vi "Set Timeout Trigger.vi"(8 "error in (no error)":errorcluster, 10 "Trigger Settings":T1, 11 "PXIe5105 in":refnum<class "PXIe5105.lvclass">) -> (0 "error out":errorcluster, 3 "PXIe5105 out":refnum<class "PXIe5105.lvclass">)   [LabVIEW 2018, in "PXIe5105.lvlib" / "PXIe5105.lvclass"]
doc: "This Override is used to configure a TimeOut Trigger."
uses:
  PXIe5105.lvclass
  PPLs/Oscilloscope/Parent/Oscilloscope.lvlibp/Custom Controls/Timeout Trigger Settings.ctl
  PPLs/Oscilloscope/Parent/Oscilloscope.lvlibp/Custom Controls/Analog Channels.ctl
  PPLs/Oscilloscope/Parent/Oscilloscope.lvlibp/Custom Controls/Trigger Mode.ctl
  PPLs/Oscilloscope/Parent/Oscilloscope.lvlibp/Custom Controls/Trigger Polarity.ctl
  <instrlib>/niScope/Controls/niScope trigger coupling.ctl
  <instrlib>/niScope/Controls/niScope trigger slope.ctl
  PXIe5105.lvclass/PXIe5105.ctl
  <instrlib>/niScope/Configure/Trigger/niScope Configure Trigger Edge.vi
  PPLs/Oscilloscope/Parent/Oscilloscope.lvlibp
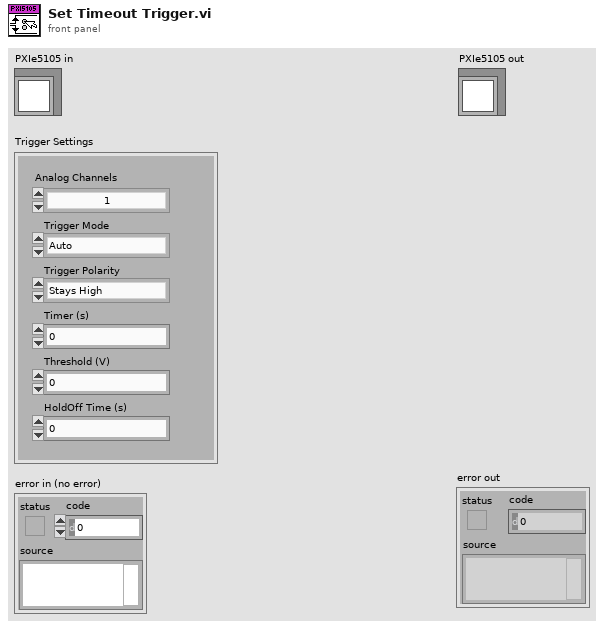
[diagram p1: front panel]
types:
  T1 = typedef "Oscilloscope.lvlibp/Timeout Trigger Settings.ctl" = cluster{"Analog Channels":T2, "Trigger Mode":T3, "Trigger Polarity":T4, "Timer (s)":dbl, "Threshold (V)":dbl, "HoldOff Time (s)":dbl}
  T2 = typedef "Oscilloscope.lvlibp/Analog Channels.ctl" = enum16{"1", "2", "3", "4", "5", "6", "7", "8", "9", "10", "11", "12", "13", "14", "15", "16"}
  T3 = typedef "Oscilloscope.lvlibp/Trigger Mode.ctl" = enum16{"Auto", "Normal"}
  T4 = typedef "Oscilloscope.lvlibp/Trigger Polarity.ctl" = enum16{"Stays High", "Stays Low", "Either"}
  T5 = typedef "niScope trigger coupling.ctl" = u16
  T6 = typedef "niScope trigger slope.ctl" = i32
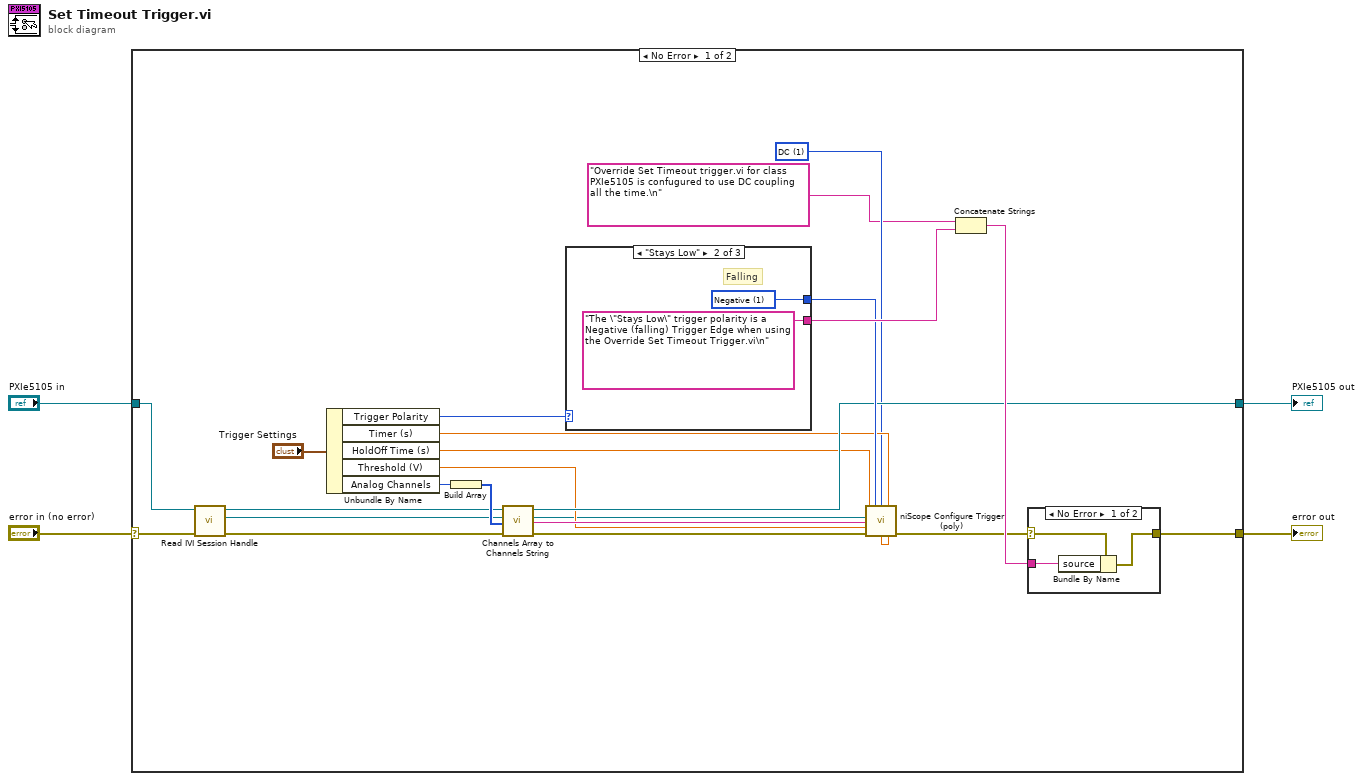
[diagram p0: block diagram]
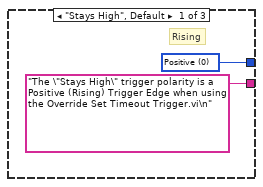
[diagram p3: hidden frame]
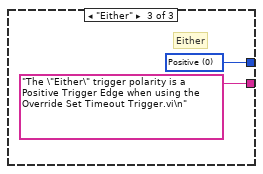
[diagram p4: hidden frame]
diagram:
  n1 = case shown="No Error" "error in (no error)" {
    selector: "error in (no error)" -> [w8 w38]
    tunnel: [w19 w38] -> w3
    tunnel: [w18 w37] -> w2
    tunnel: "PXIe5105 in" -> [w9 w37]
    frame No Error {
      w12 = T5 1 items=["AC"=0, "DC"=1, "HF Reject"=3, "LF Reject"=4, "AC Plus HF Reject"=1001] ("trigger coupling")
      n2 = call "Read IVI Session Handle.vi"("error in (no error)"=w8, "PXIe5105 in"=w9) -> ("error out"=w5:errorcluster, "IVI Session Handle"=w6:refnum<k15>, "PXIe5105 out"=w7:refnum<class "PXIe5105.lvclass">)  [unwired: 7 in]
      n3 = Unbundle By Name("Trigger Settings") -> ("Trigger Polarity"=w11:T4, "Timer (s)"=w14:dbl, "HoldOff Time (s)"=w15:dbl, "Threshold (V)"=w13:dbl, "Analog Channels"=w16:T2)
      n4 = Build Array(w16) -> (w21:T2[])
      n5 = call "Channels Array to Channels String.vi"("error in (no error)"=w5, "Channel(s) Array"=w21, "PXIe5105 in"=w7) -> ("error out"=w23:errorcluster, "Channels String"=w22:string, "PXIe5105 out"=w18:refnum<class "PXIe5105.lvclass">)  [unwired: 6 in]
      n6 = case shown="\"Stays Low\"" w11 {
        tunnel: [w32 w34 w36] -> w20
        tunnel: ["The \"Stays High\" trigger polarity is a Positive (Rising) Trigger Edge when using the Override Set Timeout Trigger.vi\n" "The \"Stays Low\" trigger polarity is a Negative (falling) Trigger Edge when using the Override Set Timeout Trigger.vi\n" "The \"Either\" trigger polarity is a Positive Trigger Edge when using the Override Set Timeout Trigger.vi\n"] -> w25
        frame "Stays High", Default {
          w32 = T6 0 items=["Positive", "Negative"] ("trigger slope")
          # "Rising"
        }
        frame "Stays Low" {
          w34 = T6 1 items=["Positive", "Negative"] ("trigger slope")
          # "Falling"
        }
        frame "Either" {
          w36 = T6 0 items=["Positive", "Negative"] ("trigger slope")
          # "Either"
        }
      }
      n7 = call-poly <instrlib>:"niScope Configure Trigger (poly).vi"("instrument handle"=w6, "trigger slope"=w20, "trigger coupling"=w12, "trigger source"=w22, "trigger level"=w13, "error in"=w23, "trigger holdoff"=w15, "trigger delay"=w14) -> ("error out"=w24:errorcluster)  [unwired: 6 in, 1 out]
      n8 = Concatenate Strings("Override Set Timeout trigger.vi for class PXIe5105 is confugured to use DC coupling all the time.\n" ("string"), w25) -> (w26:string)
      n9 = case shown="No Error" w24 {
        selector: w24 -> [w29 w30]
        tunnel: w26 -> [w28 _]
        tunnel: [w27 w30] -> w19
        frame No Error {
          n10 = Bundle By Name(cluster=w29, "source"=w28) -> (w27:errorcluster)
        }
        frame Error {
        }
      }
    }
    frame Error {
    }
  }
  "error out" <- w3
  "PXIe5105 out" <- w2
